vi "Teleop.vi"(10 "Match Info":T1={"Autonomous Elapsed Seconds"=0.0, "TeleOp Elapsed Seconds"=0.0, "Disabled Elapsed Seconds"=0.0, "Visited Autonomous"=FALSE, "Visited TeleOp"=FALSE, "Visited Disabled"=FALSE, "Autonomous Settings"={"Autonomous Style"=enum."Independent", "VI Refnum"=refnum}}, 11 "Call Context":T2) -> ()   [LabVIEW 2013]
doc: "This VI is called for each TeleOp packet received from the DS where the robot is not disabled. It is often used to read from the joysticks and update I/O or to update setpoints for timed control loops. It should complete and return within 20 milliseconds or it may miss DS packets."
uses:
  <vilib>/Rock Robotics/WPI/DriverStation/WPI_DriverStationDerivedRobotMode.ctl
  <vilib>/Rock Robotics/WPI/DriverStation/WPI_DriverStationMatch Info.ctl
  Robot Global Data.vi
  <vilib>/Rock Robotics/WPI/Joystick/WPI_JoystickGetSetRefNum.vi
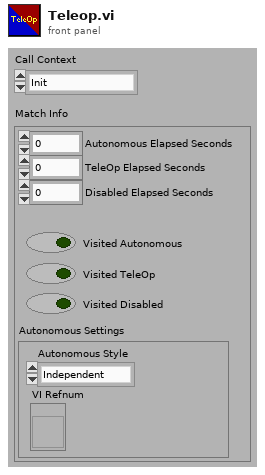
[diagram p1: front panel]
types:
  T1 = typedef "WPI_DriverStationMatch Info.ctl" = cluster{"Autonomous Elapsed Seconds":dbl, "TeleOp Elapsed Seconds":dbl, "Disabled Elapsed Seconds":dbl, "Visited Autonomous":bool, "Visited TeleOp":bool, "Visited Disabled":bool, "Autonomous Settings":cluster{"Autonomous Style":enum16{"Iterative", "Independent"}, "VI Refnum":refnum<vi>}}
  T2 = typedef "WPI_DriverStationDerivedRobotMode.ctl" = enum16{"Init", "Execute", "Stop"}
  T3 = typedef "WPI_JoystickDevRef.ctl" = cluster{"Device":T4}
  T4 = typedef "WPI_JoystickDeviceEnum.ctl" = enum16{"USB 1", "USB 2", "USB 3", "USB 4", "Kinect 1", "Kinect 2"}
  T5 = typedef "WPI_JoystickButtonState.ctl" = cluster{"Button 1":bool, "Button 2":bool, "Button 3":bool, "Button 4":bool, "Button 5":bool, "Button 6":bool, "Button 7":bool, "Button 8":bool, "Button 9":bool, "Button 10":bool, "Button 11":bool, "Button 12":bool}
  T6 = cluster{"axis 1 (x)":dbl, "axis 2 (y)":dbl, "axis 3 (throttle)":dbl, "axis 4":dbl, "axis 5":dbl, "axis 6":dbl}
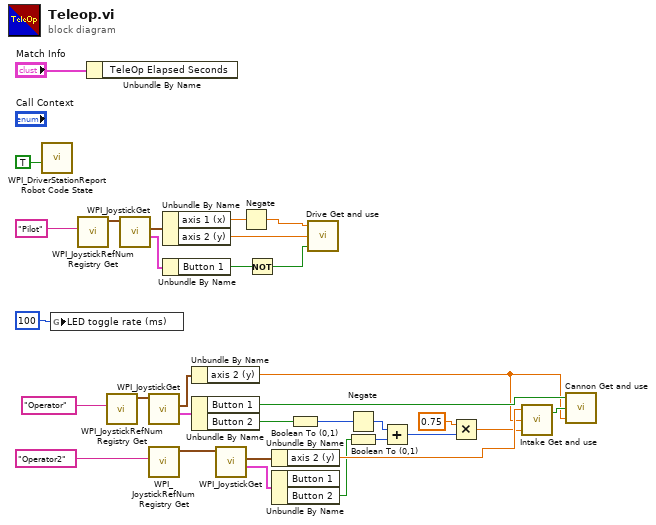
[diagram p0: block diagram]
diagram:
  n1 = call <vilib>:"WPI_DriverStationReport Robot Code State.vi"("TeleOp"=TRUE ("Autonomous")) -> ()  [unwired: 10 in, 1 out]
  n2 = global write "Robot Global Data.vi" "LED toggle rate (ms)"(u32 100 ("LED ms toggle rate")) -> ()
  n3 = call <vilib>:"WPI_JoystickRefNum Registry Get.vi"("refnum name"="Pilot") -> ("JoystickDevRef"=w26:T3)  [unwired: 9 in, 1 out]
  n4 = Unbundle By Name("Match Info") -> ()  [unwired: 1 out]
  n5 = call <vilib>:"WPI_JoystickRefNum Registry Get.vi"("refnum name"="Operator") -> ("JoystickDevRef"=w5:T3)  [unwired: 9 in, 1 out]
  n6 = call <vilib>:"WPI_JoystickGet.vi"("JoystickDevRef"=w26) -> ("Buttons"=w24:T5, "Axes"=w25:T6)  [unwired: 4 in, 1 out]
  n7 = call <vilib>:"WPI_JoystickGet.vi"("JoystickDevRef"=w5) -> ("Buttons"=w3:T5, "Axes"=w4:T6)  [unwired: 4 in, 1 out]
  n8 = call <vilib>:"WPI_JoystickRefNum Registry Get.vi"("refnum name"="Operator2") -> ("JoystickDevRef"=w13:T3)  [unwired: 9 in, 1 out]
  n9 = Unbundle By Name(w25) -> ("axis 1 (x)"=w22:dbl, "axis 2 (y)"=w29:dbl)
  n10 = Unbundle By Name(w24) -> ("Button 1"=w23:bool)
  n11 = Unbundle By Name(w4) -> ("axis 2 (y)"=w15:dbl)
  n12 = Unbundle By Name(w3) -> ("Button 1"=w19:bool, "Button 2"=w2:bool)
  n13 = call <vilib>:"WPI_JoystickGet.vi"("JoystickDevRef"=w13) -> ("Buttons"=w11:T5, "Axes"=w12:T6)  [unwired: 4 in, 1 out]
  n14 = Negate(x=w22) -> (-x=w30:dbl)
  n15 = Not(x=w23) -> (.not. x?=w28:bool)
  n16 = Unbundle By Name(w12) -> ("axis 2 (y)"=w18:dbl)
  n17 = Unbundle By Name(w11) -> ("Button 2"=w1:bool)  [unwired: 1 out]
  n18 = Boolean To (0,1)(Boolean=w2) -> (0, 1=w6:i16)
  n19 = call "Drive Get and use.vi"("Slow Drive"=w28, "Y - Axis"=w29, "X - Axis"=w30) -> ()
  n20 = Negate(x=w6) -> (-x=w7:i16)
  n21 = Boolean To (0,1)(Boolean=w1) -> (0, 1=w8:i16)
  n22 = Add(x=w7, y=w8) -> (x+y=w10:i16)
  n23 = Multiply(x=0.75, y=w10) -> (x*y=w17:dbl)
  n24 = call "Intake Get and use.vi"("TakeBall"=w17, "Cannon vbus"=w15, "Upper Claw"=w18) -> ("InTake Max"=w16:bool)  [unwired: 1 out]
  n25 = call "Cannon Get and use.vi"("Move"=w15, "InTake Max"=w16, "Fire"=w19) -> ()  [unwired: 1 out]
